vi "read-image.vi"(9 "calibration":i32, 10 "pos":i32, 11 "ir_file_handler":u64) -> (2 "pixels":u16[][](array[numeric]), 3 "ir_file_handler":u64)   [LabVIEW 2011, in "librir.lvlib"]
uses:
  librir.lvlib
  libs/video_io.dll
panel:
  out "return value":i16
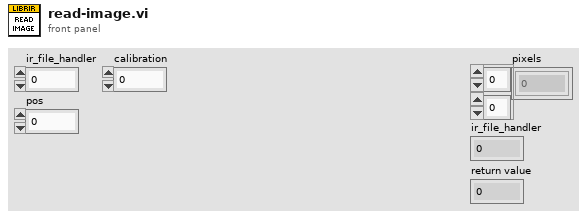
[diagram p1: front panel]
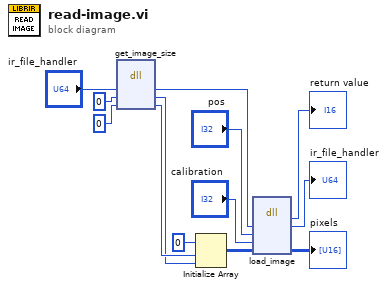
[diagram p0: block diagram]
diagram:
  n1 = dll-call lib="G:/librir/src/labview/libs/video_io.dll" fn="get_image_size"("ir_file_handler"="ir_file_handler", "width"=0, "height"=0) -> ("ir_file_handler"=w10:u64, "width"=w6:i32, "height"=w7:i32)  [unwired: 4 in, 2 out]
  n2 = Initialize Array(u16 0, w7, w6) -> (w5:u16[][])
  n3 = dll-call lib="G:/librir/src/labview/libs/video_io.dll" fn="load_image"("ir_file_handler"=w10, "pos"="pos", "calibration"="calibration", "pixels"=w5) -> ("return value"=→"return value":i16, "ir_file_handler"=→"ir_file_handler":u64, "pixels"=→"pixels":u16[][])  [unwired: 5 in, 2 out]
